vi "Latch_Switch.vi"(1 "Reset":bool, 2 "In":bool) -> (0 "Out":bool)   [LabVIEW 2015]
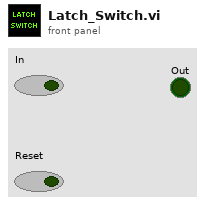
[diagram p1: front panel]
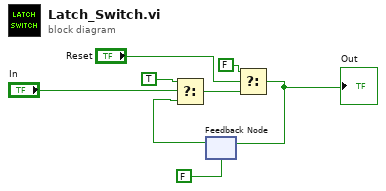
[diagram p0: block diagram]
diagram:
  n1 = feedback #1(FALSE) -> (w2:bool)
  n2 = Select(t=TRUE, s="In", f=w2) -> (s? t:f=w8:bool)
  n3 = Select(t=FALSE, s="Reset", f=w8) -> (s? t:f=w3:bool)
  "Out" <- w3
  n4 = feedback-in #1(w3) -> ()
